vi "Add to log.vi"(7 "Rewerse":bool, 10 "String in":string, 11 "Log":string) -> (3 "String out":string)   [LabVIEW 2021]
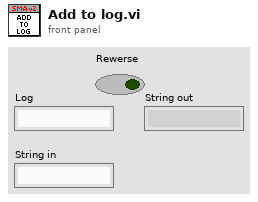
[diagram p1: front panel]
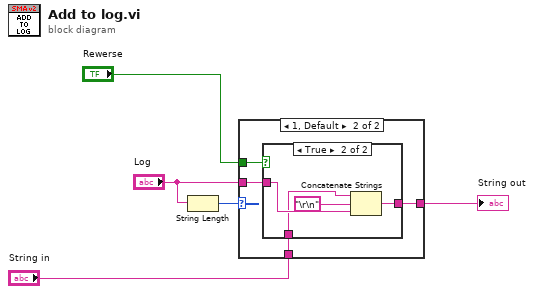
[diagram p0: block diagram]
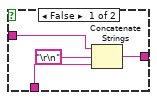
[diagram p3: hidden frame]
diagram:
  n1 = String Length(string="Log") -> (length=w4:i32)
  n2 = case shown="1, Default" w4 {
    tunnel: [w6 w10] -> w2
    tunnel: "String in" -> [w6 w9]
    tunnel: "Log" -> [_ w8]
    tunnel: "Rewerse" -> [_ w7]
    frame 0 {
    }
    frame 1, Default {
      n3 = case shown="True" w7 {
        tunnel: [w14 w15] -> w10
        tunnel: w9 -> [w13 w16]
        tunnel: w8 -> [w11 w17]
        frame False {
          n4 = Concatenate Strings(w11, "\r\n", w13) -> (w14:string)
        }
        frame True {
          n5 = Concatenate Strings(w16, "\r\n", w17) -> (w15:string)
        }
      }
    }
  }
  "String out" <- w2
